vi "Initialize GPS.vi"(8 "error in (no error)":errorcluster, 11 "Device ID":T1) -> (0 "error out":errorcluster, 2 "Sensor Error":i32, 3 "Garmin GPS Series out":refnum<class "Garmin GPS Series.lvclass">)   [LabVIEW 2012, in "UniCyRO.lvlib" / "UniCyRO_Host_Sim.lvclass"]
uses:
  UniCyRO_Host_Sim.lvclass
  <vilib>/robotics/Simulator/Engine/ctl/DeviceID.ctl
  <instrlib>/Garmin GPS Series/HAIOL/Garmin GPS Series.lvclass
  <vilib>/robotics/Utilities/NI_Robotics Utilities.lvlib
  <instrlib>/Garmin GPS Series/HAIOL/Simulator/Garmin GPS Series Simulator.lvclass
  <vilib>/robotics/Simulator/NI_Robotics_Simulator.lvlib
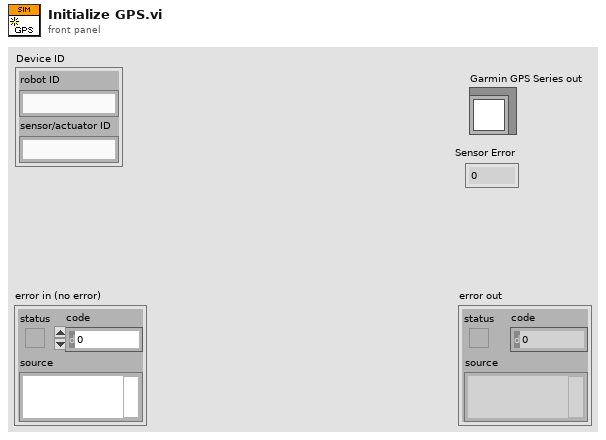
[diagram p1: front panel]
types:
  T1 = typedef "NI_Robotics_Simulator.lvlib/DeviceID.ctl" = cluster{"robot ID":string, "sensor/actuator ID":string}
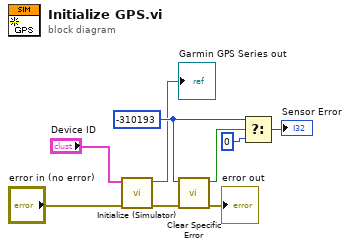
[diagram p0: block diagram]
diagram:
  w6 = -310193 ("code")
  n1 = call <instrlib>:"Initialize (Simulator).vi"("error in (no error)"="error in (no error)", "Device ID"="Device ID") -> ("error out"=w3:errorcluster, "Garmin GPS Series out"=→"Garmin GPS Series out":refnum<class "Garmin GPS Series.lvclass">)  [unwired: 8 in]
  n2 = call <vilib>:"Clear Specific Error.vi"("error in (no error)"=w3, "code"=w6) -> ("error out"=→"error out":errorcluster, "code found?"=w7:bool)  [unwired: 7 in, 1 out]
  n3 = Select(t=w6, s=w7, f=0) -> (s? t:f=→"Sensor Error":i32)
